vi "Read_Temp_Data_Log.vi"(8 "error in (no error)":errorcluster, 11 "DataLogPath":path) -> (0 "error out":errorcluster, 2 "Data":string[][](array[string]))   [LabVIEW 2012]
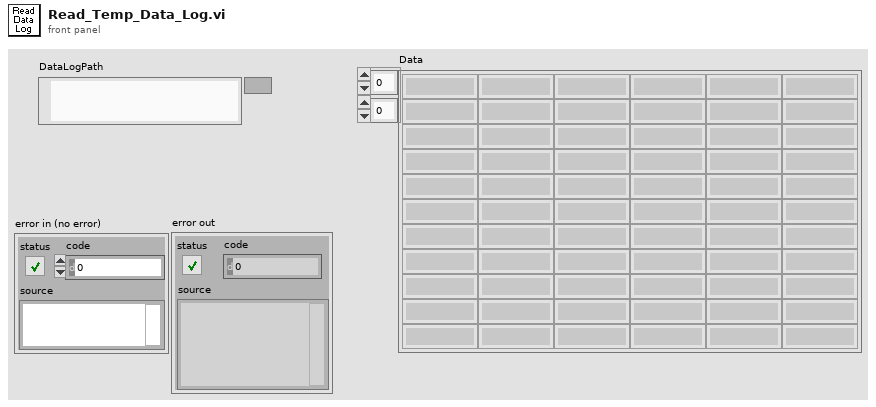
[diagram p1: front panel]
types:
  T1 = enum16{"deny read/write", "deny write-only", "deny none"}
  T2 = enum16{"open", "replace", "create", "open or create", "replace or create", "replace or create with confirmation"}
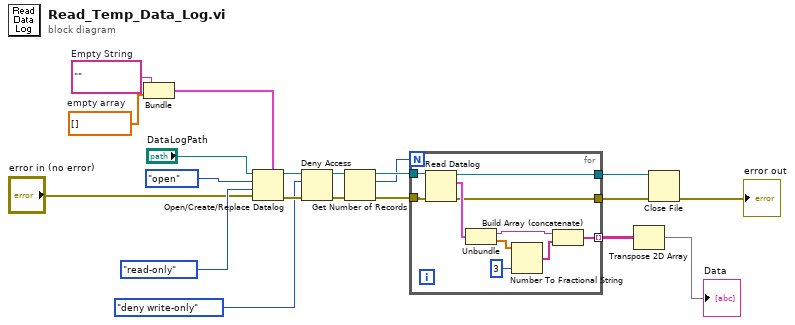
[diagram p0: block diagram]
diagram:
  w17 = ""  # Empty String
  w18 = sgl[] []  # empty array
  n1 = Bundle(w17, "empty array"=w18) -> (w19:cluster{string, "empty array":sgl[]})  [unwired: 1 out]
  n2 = Open/Create/Replace Datalog(5:w19, 8:"error in (no error)", 9:enum16{"read/write", "read-only", "write-only"}."read-only" ("access (0:read/write)"), 10:T2."open" ("operation (0:open)"), 11:"DataLogPath") -> (0:w9:errorcluster, 3:w7:refnum<k1>)  [unwired: 2 out]
  n3 = Deny Access(4:w9, 6:T1."deny write-only" ("deny mode (0:deny read/write)"), 7:w7) -> (0:w8:errorcluster, 3:w6:refnum<k1>)
  n4 = Get Number of Records(4:w8, 7:w6) -> (0:w15:errorcluster, 2:w13:i64, 3:w14:refnum<k1>)
  n5 = for {
    N: w13 -> [_]
    tunnel: [w29] -> w2 mode=indexing
    tunnel: w15 -> [w28]
    tunnel: [w26] -> w11
    tunnel: w14 -> [w25]
    tunnel: [w24] -> w12
    n6 = Read Datalog(4:w28, 7:w25) -> (0:w26:errorcluster, 2:w27:cluster{string, "empty array":sgl[]}, 3:w24:refnum<k1>)  [unwired: 1 out]
    n7 = Unbundle(w27) -> (w30:string, "empty array"=w23:sgl[])
    n8 = Number To Fractional String(number=w23, precision (6)=i16 3) -> (F-format string=w22:string[])  [unwired: 2 in]
    n9 = Build Array (concatenate)(w30, w22) -> (w29:string[])
  }
  n10 = Transpose 2D Array(2D array=w2) -> (transposed array=→"Data":string[][])
  n11 = Close File(refnum=w12, error in=w11) -> (error out=→"error out":errorcluster)  [unwired: 1 out]
